vi "Actor Core.vi"(8 "error in":errorcluster, 11 "Waiting Dialog View in":refnum<class "Waiting Dialog View.lvclass">) -> (0 "error out":errorcluster, 3 "Actor out":refnum<class "Actor.lvclass">)   [LabVIEW 2020, in "Waiting Dialog View.lvlib" / "Waiting Dialog View.lvclass"]
doc: "(<B>Filename</B>: Actor Framework.lvlib:Actor.lvclass:Actor Core.vi)\n\nReceives messages to the actor, reacts to them, and initiates any error handling that may shut the actor down.\n\nDescendant classes may override this VI to append parallel tasks for the actor to complete while it handles messages. Overrides use the Call Parent Method node."
uses:
  Waiting Dialog View.lvclass
  <vilib>/ActorFramework/Actor/Actor.lvclass
  <vilib>/Utility/miscctls.llb/LVPositionTypeDef.ctl
  <vilib>/ActorFrameworkMVC/Abstract View/Abstract View/Abstract View.lvclass
panel:
  out "Message":string="Printing, please wait a moment."
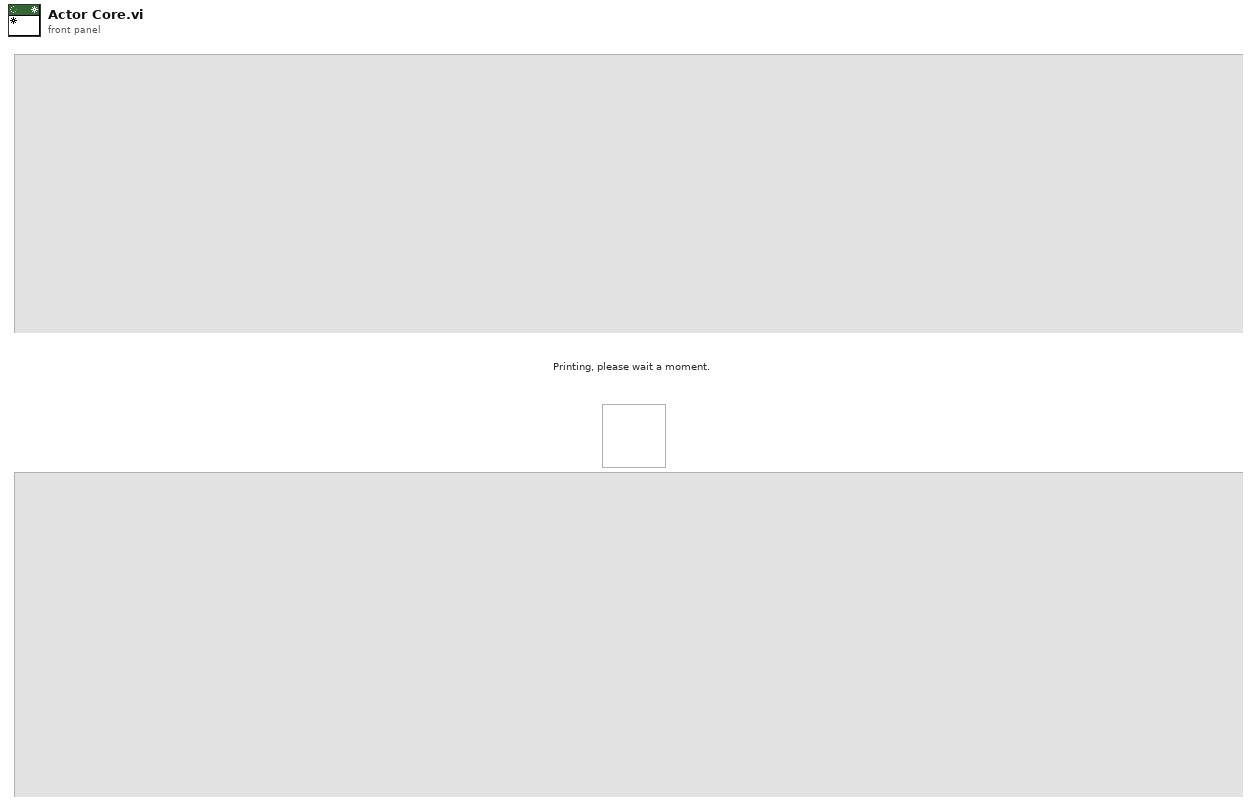
[diagram p1: front panel]
types:
  T1 = typedef "LVPositionTypeDef.ctl" = cluster{"Left":i32, "Top":i32}
  T2 = typedef "LVRectTypeDef.ctl" = cluster{"Left":i16, "Top":i16, "Right":i16, "Bottom":i16}
  T3 = typedef "LVBoundsTypeDef.ctl" = cluster{"Width":u32, "Height":u32}
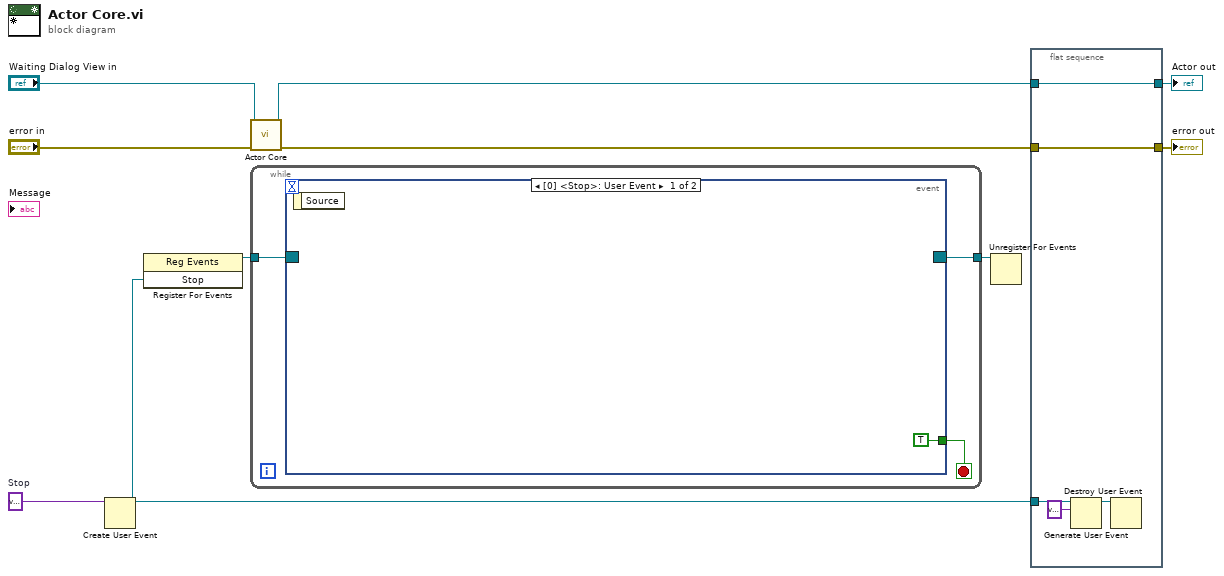
[diagram p0: block diagram]
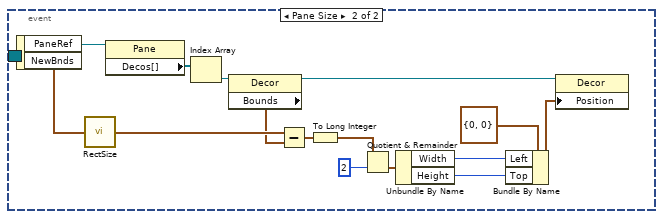
[diagram p2: hidden frame]
diagram:
  w8 = variant  # Stop
  n1 = Create User Event(user event datatype=w8) -> (user event=w1:refnum<user-event>)  [unwired: 1 in, 1 out]
  n2 = register-events(w1) -> (reference out=w9:refnum<event-registration>)  [unwired: 2 in, 1 out]
  n3 = call-parent "Actor Core.vi"("error in"="error in", "Abstract View in"="Waiting Dialog View in") -> ("error out"=w4:errorcluster, "Actor out"=w6:refnum<class "Actor.lvclass">)  [unwired: 8 in]
  n4 = while {
    tunnel: w9 -> [w13]
    tunnel: [w12] -> w7
    stop <- w11 stop-if-true
    n5 = event shown="[0] <Stop>: User Event" {
      selector: w13 -> [_ _]
      dyn-events: [_ _] -> w12
      timeout: _ -> [_ _]
      tunnel: [TRUE _] -> w11
      event User Event {
        n6 = event-data() -> ()  [unwired: 1 in, 1 out]
      }
      event Pane Size {
        n7 = event-data() -> ("PaneRef"=w16:refnum<vi>, "NewBnds"=w15:T2)  [unwired: 1 in]
        n8 = call <vilib>:"RectSize.vi"("rect"=w15) -> ("point"=w24:cluster{"x":i16, "y":i16})
        n9 = property class="Pane"(reference=w16) -> ("Decos[]"=w29:refnum<vi>[])  [unwired: 1 in, 2 out]
        n10 = Index Array(array=w29) -> (element=w28:refnum<vi>)  [unwired: 1 in]
        n11 = property class="Decor"(reference=w28) -> (reference out=w27:refnum<vi>, "Bounds"=w19:T3)  [unwired: 1 in, 1 out]
        n12 = Subtract(x=w24, y=w19) -> (x-y=w21:T3)
        n13 = To Long Integer(number=w21) -> (32bit integer=w18:cluster{"Width":i32, "Height":i32})
        n14 = Quotient & Remainder(x=w18, y=2) -> (floor(x/y)=w20:cluster{"Width":i32, "Height":i32})  [unwired: 1 out]
        n15 = Unbundle By Name(w20) -> ("Width"=w23:i32, "Height"=w22:i32)
        n16 = Bundle By Name(cluster=T1 {"Left"=0, "Top"=0} ("Position"), "Left"=w23, "Top"=w22) -> (w17:T1)
        n17 = property class="Decor"(reference=w27, "Position"=w17) -> ()  [unwired: 1 in, 2 out]
      }
    }
  }
  n18 = Unregister For Events(event registration refnum=w7) -> ()  [unwired: 1 in, 1 out]
  n19 = flat-sequence {
    tunnel: w6 -> [w32]
    tunnel: [w32] -> w5
    tunnel: w4 -> [w31]
    tunnel: [w31] -> w3
    tunnel: w1 -> [w30]
    frame #0 {
      n20 = Generate User Event(user event=w30, event data cluster=variant ("event data")) -> (user event out=w33:refnum<user-event>)  [unwired: 2 in, 1 out]
      n21 = Destroy User Event(user event=w33) -> ()  [unwired: 1 in, 1 out]
    }
  }
  "error out" <- w3
  "Actor out" <- w5
